vi "NET_Limit_Switches.vi"(8 "Read(F) Write(T)":bool, 11 "Switches In":T1) -> (3 "Switches Out":T1)   [LabVIEW 2017]
uses:
  RoboRio Code/TypeDef/CLUSTER_Limit_Switches.ctl
  <vilib>/Rock Robotics/Network Tables/NT Read Boolean Array.vi
  <vilib>/Rock Robotics/Network Tables/NT Write Boolean Array.vi
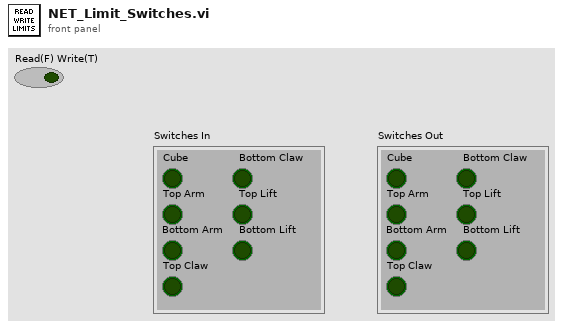
[diagram p1: front panel]
types:
  T1 = typedef "CLUSTER_Limit_Switches.ctl" = cluster{"Cube":bool, "Top Arm":bool, "Bottom Claw":bool, "Top Lift":bool, "Bottom Arm":bool, "Bottom Lift":bool, "Top Claw":bool}
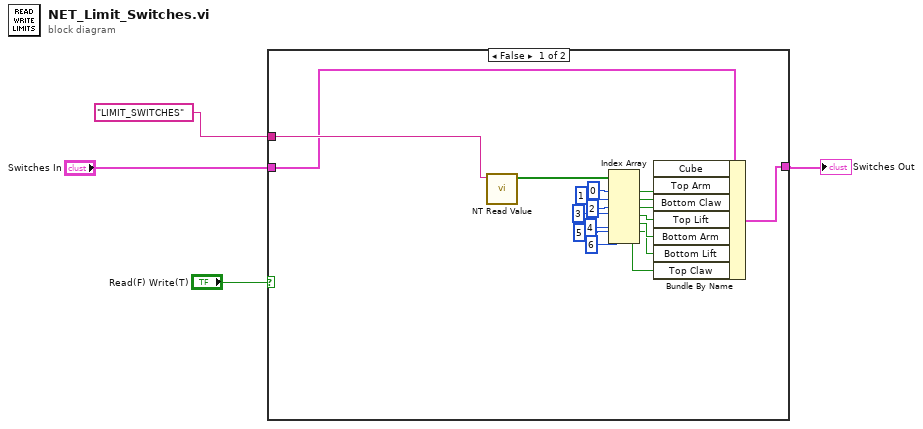
[diagram p0: block diagram]
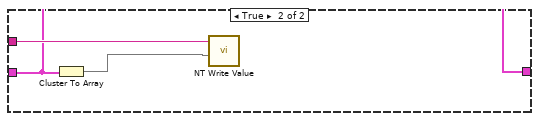
[diagram p2: hidden frame]
diagram:
  n1 = case shown="False" "Read(F) Write(T)" {
    tunnel: "LIMIT_SWITCHES" ("Name") -> [w22 w25]
    tunnel: "Switches In" -> [w13 w23]
    tunnel: [w9 w23] -> w1
    frame False {
      n2 = call-poly <vilib>:"NT Read Value.vi"("Name"=w22) -> ("Boolean Array"=w21:bool[])  [unwired: 9 in, 1 out]
      n3 = Index Array(array=w21, index #1=0 ("index"), index #2=1 ("index"), index #3=2 ("index"), index #4=3 ("index"), index #5=4 ("index"), index #6=5 ("index"), index #7=6 ("index")) -> (element #1=w14:bool, element #2=w12:bool, element #3=w11:bool, element #4=w10:bool, element #5=w7:bool, element #6=w6:bool, element #7=w5:bool)
      n4 = Bundle By Name(cluster=w13, "Cube"=w14, "Top Arm"=w12, "Bottom Claw"=w11, "Top Lift"=w10, "Bottom Arm"=w7, "Bottom Lift"=w6, "Top Claw"=w5) -> (w9:T1)
    }
    frame True {
      n5 = Cluster To Array(cluster=w23) -> (array=w24:bool[])
      n6 = call-poly <vilib>:"NT Write Value.vi"("Boolean Array"=w24, "Name"=w25) -> ()  [unwired: 9 in, 1 out]
    }
  }
  "Switches Out" <- w1
